vi "nirviMemRead.vi"(0 "Address":u16) -> (1 "Data":u16, 2 "Failure":bool)   [LabVIEW 2020]
doc: "<B>LabVIEW no longer supports this VI. Use the Memory Read function configured for a memory item instead.</B>\n\nReads from memory available on the FPGA. There are 16 KB of memory available, organized as 8 K x 16 bits. Use the Memory Read VI in conjunction with the Memory Write VI.\n\nIf you use the Memory Read VI in a single-cycle Timed Loop, wire the outputs directly to uninitialized shift registers or feedback nodes. The Memory Read VI takes an entire clock cycle to execute. You cannot use memory to transfer data among multiple clock domains."
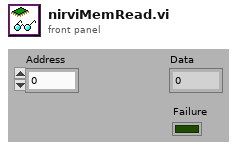
[diagram p1: front panel]
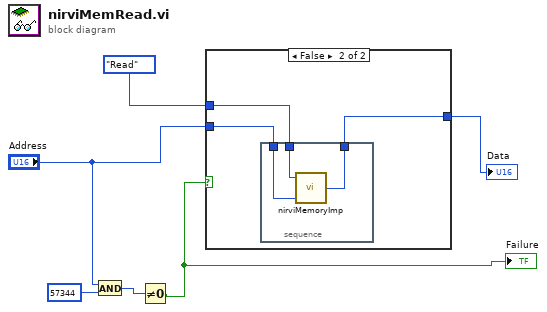
[diagram p0: block diagram]
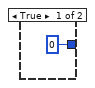
[diagram p2: hidden frame]
diagram:
  n1 = And(x="Address", y=u16 57344) -> (x .and. y?=w6:u16)
  n2 = Not Equal To 0?(x=w6) -> (x != 0?=w1:bool)
  "Failure" <- w1
  n3 = case shown="False" w1 {
    tunnel: enum16{"Read", "Write"}."Read" -> [_ w10]
    tunnel: "Address" -> [_ w9]
    tunnel: [u16 0 ("Data 2") w8] -> w3
    frame True {
    }
    frame False {
      n4 = stacked-sequence {
        tunnel: w10 -> [w13]
        tunnel: w9 -> [w12]
        tunnel: [w11] -> w8
        frame #0 {
          n5 = call <vilib>:"nirviMemoryImp.vi"("Address"=w12, "Enum"=w13) -> ("Data 2"=w11:u16)  [unwired: 1 in]
        }
      }
    }
  }
  "Data" <- w3
